vi "FPGA1483V1_0.vi"() -> ()   [LabVIEW 2013]
doc: "This is the FPGA VI for the 10-Tap 8-Bit Camera with DRAM example. This example demonstrates how to acquire images from a 10-tap, 8-bit, extended configuration, Camera Link camera and transfer the images to the host. This example supports area scan and line scan cameras for both continuous and finite acquisitions.\n\nThis example also demonstrates the use of DRAM as a frame buffer for very high speed acquisitions. Data packing and flow-control are also employed to maximize use of the available DRAM and FIFOs in terms of both memory space and performance.\n\nAdditionally, the example demonstrates the serial server, which allows third-party camera configuration utilities to communicate with the camera using the Camera Link serial interface while this VI is running."
uses:
  <vilib>/Platform/TimedLoop/XDataNode/timing_clust.ctl
  <vilib>/Platform/TimedLoop/XDataNode/nitl_modes.ctl
  <vilib>/Platform/TimedLoop/XDataNode/wakeup.ctl
  <vilib>/rvi/eio/common/nirviEmuTemplateMethod_errors.vi
  <vilib>/rvi/Emulation/niFpgaSctlEmulationGetInTimedLoop.vi
  <vilib>/rvi/Emulation/niFpgaEmulationReportErrorSimple.vi
  <vilib>/rvi/Emulation/niFpgaGetClockAttributes.vi
  <vilib>/rvi/Emulation/niFpgaCriticalErrorInLSC.vi
  Common/CL Data to Pixels/10 Tap 8-Bit.vi
  <vilib>/rvi/interface/RandomDataEmulation/nirviRandomDataFPGAFIFO.vi
  <vilib>/rvi/interface/RandomDataEmulation/niFpgaRandomDataHandleErrors.vi
  <vilib>/rvi/FIFO/Fifo_Resource/nirvififoEmulationWriteFpgaImpl.vi
  <vilib>/rvi/DataTransferAndStorage/Container/Common/niFpgaContainerGetUniqueNameForEmu.vi
  <vilib>/rvi/FIFO/Fifo_Resource/nirvififoEmulationGetNumberOfElementsToReadFpgaImpl.vi
  <vilib>/rvi/FIFO/Fifo_Resource/nirvififoEmulationReadFpgaImpl.vi
  <vilib>/rvi/Emulation/niFpgaProcessEmulError.vi
  <vilib>/Platform/TimedLoop/XDataNode/XDataNode.xnode
  <vilib>/eio/EIONode/EIONode.xnode
  <vilib>/rvi/DataTransferAndStorage/Container/XNode/niFpgaContainer.xnode
  <vilib>/rvi/interface/RandomDataEmulation/nirviRandomDataFpgaReadWriteTemplate.vi
  <vilib>/rvi/FIFO/Fifo_Resource/nirvififoEmulationWrite.vi
  <vilib>/rvi/FIFO/Fifo_Resource/nirvififoEmulationGetNumberOfElementsToRead.vi
  <vilib>/rvi/FIFO/Fifo_Resource/nirvififoEmulationRead.vi
  <vilib>/Platform/TimedLoop/XDataNode/XDNodeRunTimeDep.lvlib
panel:
  in  "DigitalEnable":bool=TRUE
  out "auxAI1":i16
  in  "auxAO0":i16
  out "auxAI0":i16
  out "DI1":bool
  out "DI0":bool
  in  "DO1":bool
  in  "DO0":bool
  out "DevQualityStatus":u8
  out "DMAsOverflow":u16
  out "BytesperSampleChannelDMATtoHOST":u8[](array[numeric])=[12]
  out "FrameTypeDMATtoHOST":u8[](array[numeric])=[12]
  out "Platform":enum8{"FlexRIO", "cRIO", "RSeries"}(ring)
  in  "GroupEnable0":bool
  out "DMAsOverflowB":bool
  out "DevProfile":u8=1
  out "RIOAdapterCorrect":bool
  out "InsertedIOModule ID":u32=278099145
  out "ExpectedIOModule ID":u32=278099145
  in  "DebugMode":bool
  in  "SamplingRate0":u16
  out "DeviceTemp":i16=147
  in  "DataBytetoTx":i32=1 format="%x"
  in  "DAQStartStop":bool
  out "NCHperDMATtoHOST":u8[](array[numeric])=[1]
  out "FPGAVIversion":u8[](array[numeric])=[1, 1]
  out "NoOfWFGen":u8
  out "Fref":u32=100000000
  in  "ControlEnable":bool=TRUE caption="IO Module\\CL Control Enable"
  in  "Configuration":u8=2 caption="CL Config.Configuration"
  in  "SignalMapping":u8 caption="CL Config.Signal Mapping"
  in  "LineScan":bool caption="CL Config.Line Scan"
  in  "DVALHigh":bool=TRUE caption="CL Config.DVAL Active High"
  in  "LVALHigh":bool=TRUE caption="CL Config.LVAL Active High"
  in  "FVALHigh":bool=TRUE caption="CL Config.FVAL Active High"
  in  "SpareHigh":bool=TRUE caption="CL Config.Spare Active High"
  in  "Acq Control.Line Scan Height":u32
  in  "Acq Control.Frames To Acq":u32
  in  "StartDAQ":bool
  in  "StopDAQ":bool
  in  "Acq Control.Ignore DVAL":bool
  out "Acq Status.Acq In Progress":bool
  out "Acq Status.Clocks Per Line":u32
  out "Acq Status.Frames Acq'd":u32
  out "Acq Status.Lines Per Frame":u32
  out "auxDO11":bool caption="Acq Status.DMA Write Timeout"
  out "InitDone":bool
  in  "uartBaudRate":i32=1 caption="UART.Baud Rate"
  in  "uartTransmit":bool caption="UART.Transmit"
  in  "uartSetBaudRate":bool caption="UART.Set Baud Rate"
  in  "uartByteMode":bool=TRUE caption="UART.Byte Mode"
  out "uartRxReady":bool caption="auxDI1"
  out "uartBreakIndicator":bool caption="UART.Break Indicator"
  out "uartFramingError":bool caption="UART.Framing Error"
  out "uartOverrunError":bool caption="UART.Overrun Error"
  out "uartTxReady":bool caption="UART.Tx Ready"
  out "uartRxData":i32 caption="UART.Rx Data" format="%02x"
  in  "uartReceive":bool caption="UART.Receive"
  # "This terminal has not sense in this solution"
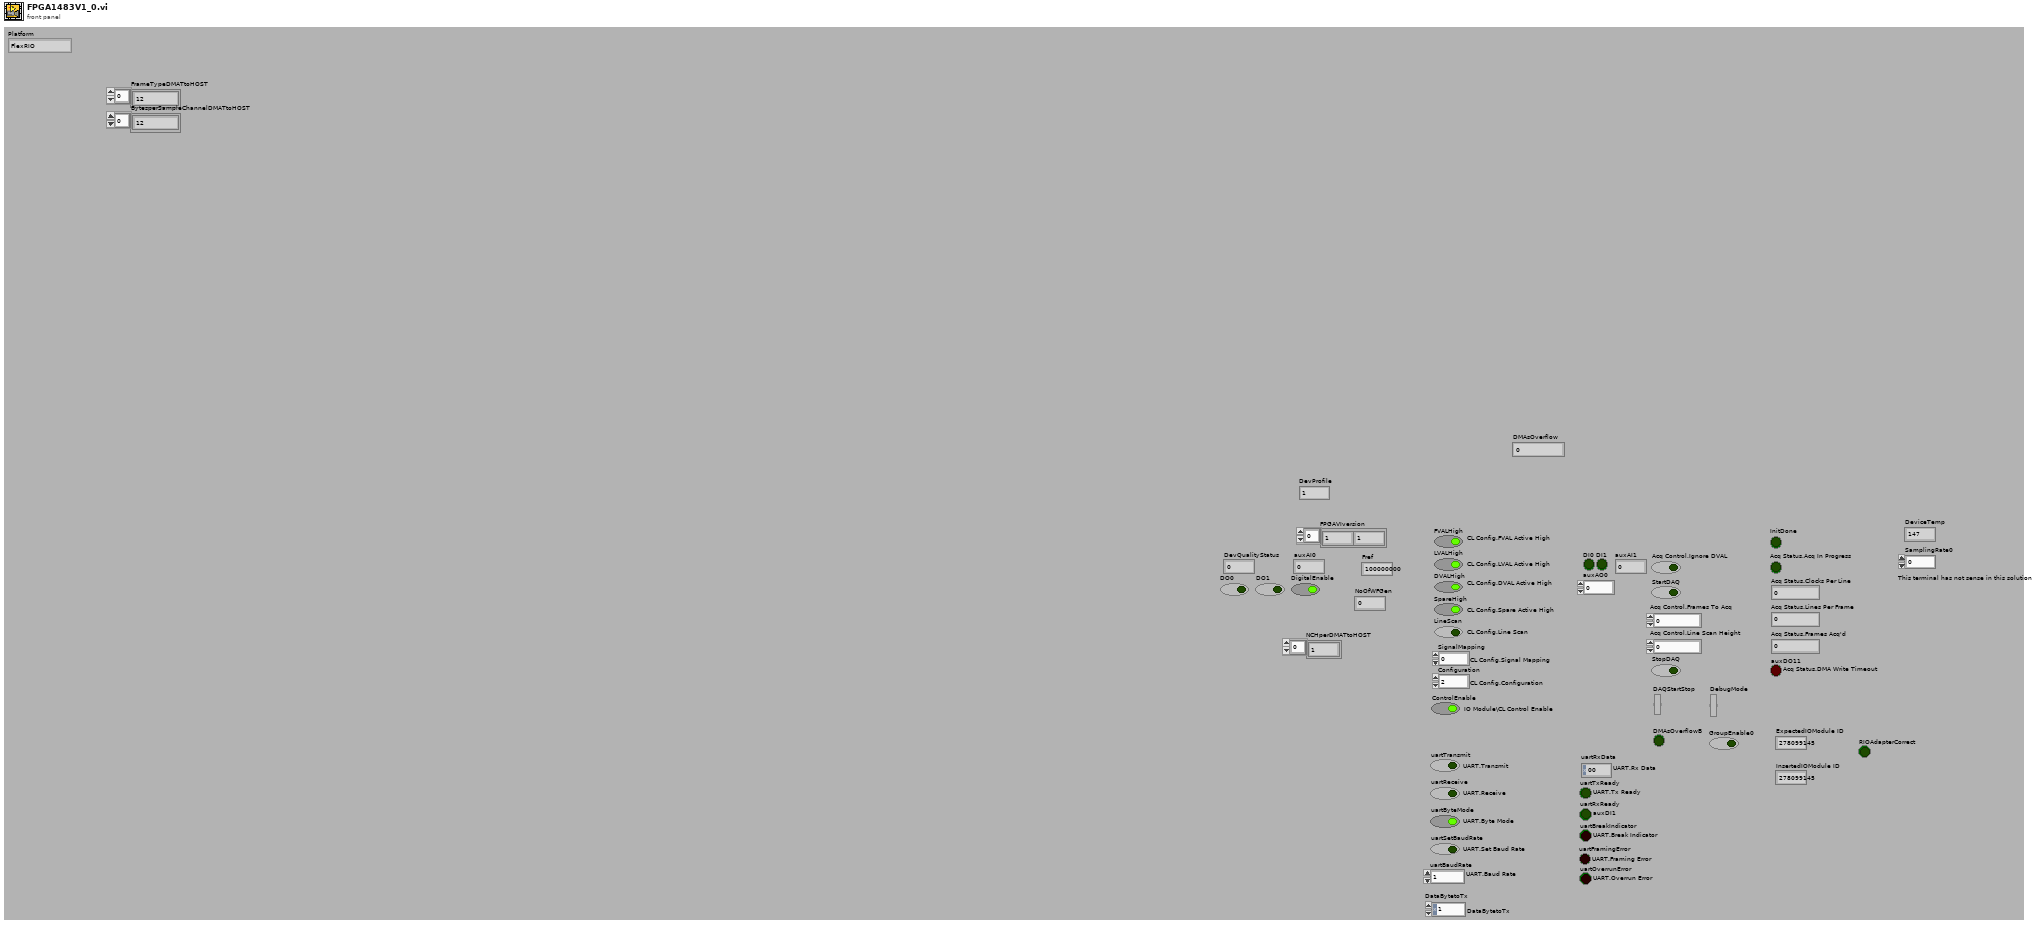
[diagram p1: front panel]
types:
  T1 = typedef "XDNodeRunTimeDep.lvlib/timing_clust.ctl" = cluster{"Expected End [f-1]":u64, "Actual End [f-1]":u64, "Finished Late? [f-1]":bool, "Expected End [i-1]":u64, "Actual End [i-1]":u64, "Finished Late? [i-1]":bool, "Expected Start [i]":u64, "Actual Start [i]":u64, "Expected Start [f]":u64, "Actual Start [f]":u64, "Source Name":string, "Structure Name":string, "Period":i64, "Deadline":i64, "Offset":i64, "Start":i64, "Priority":i32, "Timeout":i32, "Mode":T2, "Wakeup Reason":T3, "Error":errorcluster, "Source Type":string, "Secondary Source Type":string, "Global End Time":u64, "Global Start Time":u64, "Frame Duration":u64, "Iteration Duration":u64, "Assigned CPU":i32, "I/O Scan Engine Mode":u32}
  T2 = typedef "XDNodeRunTimeDep.lvlib/nitl_modes.ctl" = enum32{"No Change", "Process missed periods, maintain original phase", "Discard missed periods, maintain original phase", "Process missed periods, ignore original phase", "Discard missed periods, ignore original phase"}
  T3 = typedef "XDNodeRunTimeDep.lvlib/wakeup.ctl" = enum32{"Normal", "Aborted", "Asynchronous wakeup", "Timing source error", "Timed loop error", "Timeout"}
  T4 = cluster{"Enables Valid":bool, "Frame Valid":bool, "Line Valid":bool, "Data Valid":bool}
  T5 = enum8{"Standard", "Basler 10-tap", "Vosskühler 10-tap"}
  T6 = cluster{"Pixel 0":u8, "Pixel 1":u8, "Pixel 2":u8, "Pixel 3":u8, "Pixel 4":u8, "Pixel 5":u8, "Pixel 6":u8, "Pixel 7":u8, "Pixel 8":u8, "Pixel 9":u8}
  T7 = cluster{"Tx Data":u8[], "Transmit":bool, "Receive":bool, "Byte Mode":bool, "Set Baud Rate":bool, "Baud Rate":u8}
  T8 = cluster{"Rx Data":u8, "Turn Off Transmit":bool, "Turn Off Receive":bool, "Turn Off Set Baud Rate":bool, "Tx Ready":bool, "Rx Ready":bool, "Break Indicator":bool, "Framing Error":bool, "Overrun Error":bool}
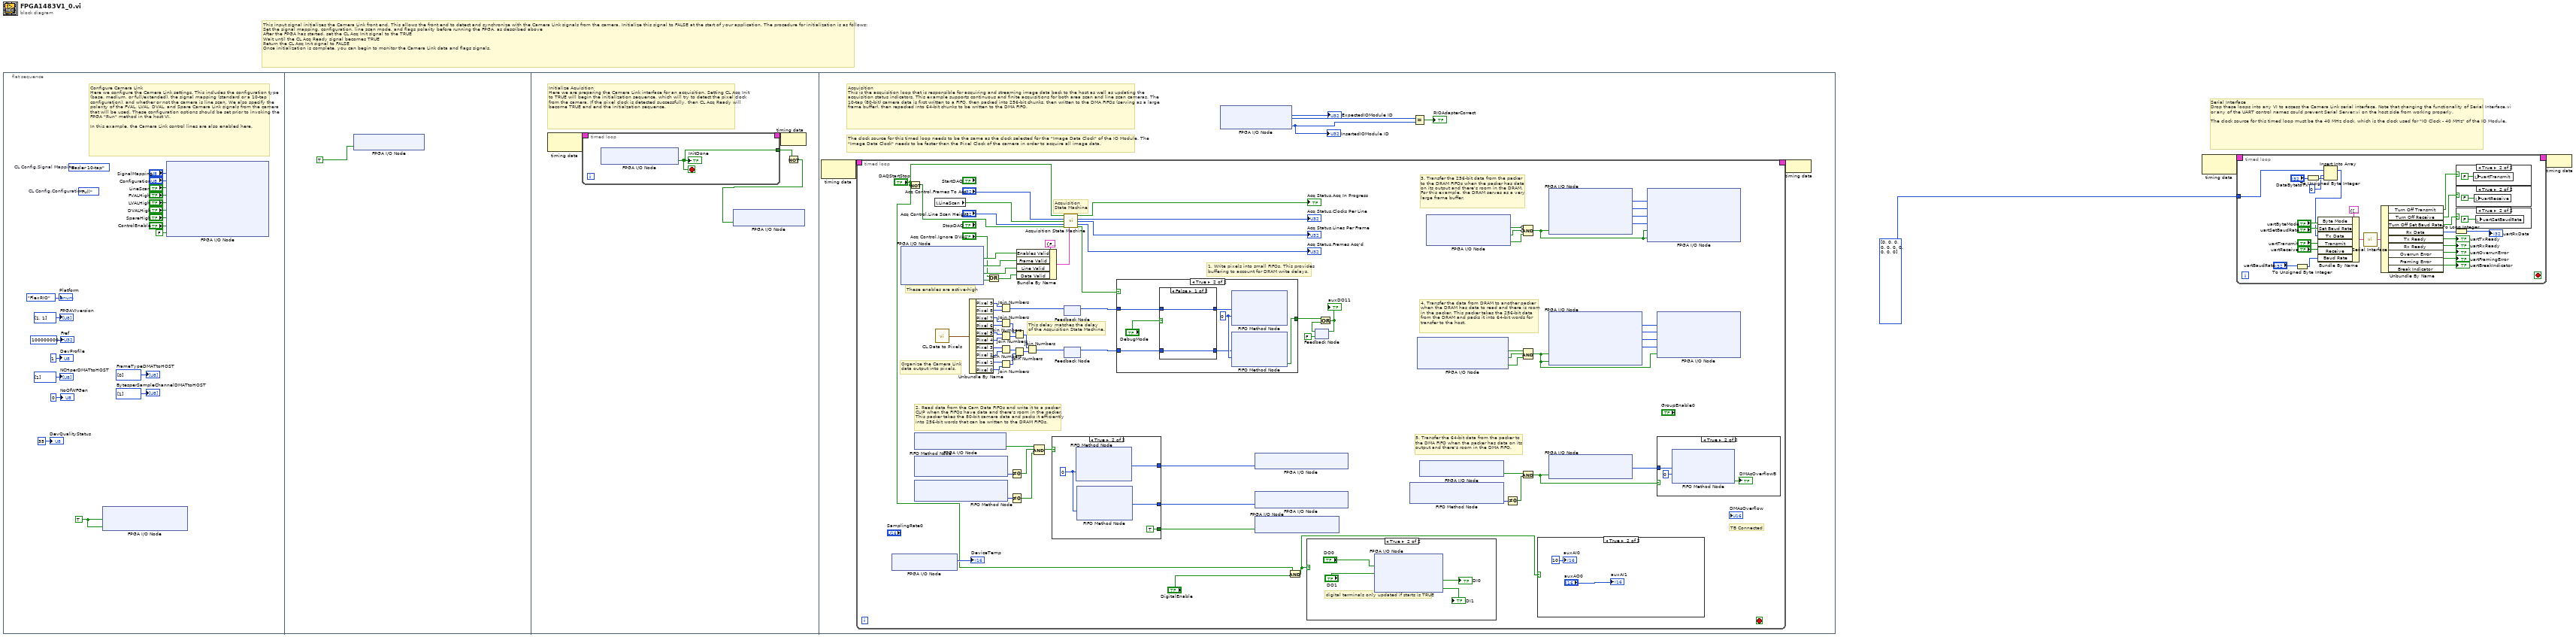
[diagram p0: block diagram]
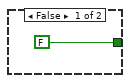
[diagram p9: hidden frame]
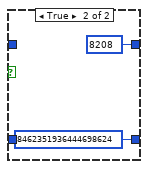
[diagram p10: hidden frame]
diagram:
  # "This input signal initializes the Camera Link front end. This allows the front end to detect and synchronize with the Camera Link signals from the camera. Initialize this signal to FALSE at the start of your application. The procedure for initialization is as follows: \nSet the signal mapping, configuration, line scan mode, and flags polarity before running the FPGA, as described above \nAfter the FPGA has started, set the CL Acq Init signal to the TRUE \nWait until the CL Acq Ready signal becomes TRUE \nReturn the CL Acq Init signal to FALSE \nOnce initialization is complete, you can begin to monitor the Camera Link data and flags signals."
  # "Serial Interface\nDrop these loops into any VI to access the Camera Link serial interface. Note that changing the functionality of Serial Interface.vi or any of the UART control names could prevent Serial Server.vi on the host side from working properly.\n\nThe clock source for this timed loop must be the 40 MHz clock, which is the clock used for \"IO Clock - 40 MHz\" of the IO Module."
  n1 = flat-sequence {
    frame #0 {
      w4 = TRUE ("IO Module\\TTL Out Enable 0")
      (unwired) T5."Basler 10-tap"  # CL Config.Signal Mapping
      (unwired) enum8{"Base", "Medium", "Full"}."Full"  # CL Config.Configuration
      # "Configure Camera Link\nHere we configure the Camera Link settings. This includes the configuration type (base, medium, or full/extended), the signal mapping (standard or a 10-tap configuration), and whether or not the camera is line scan. We also specify the polarity of the FVAL, LVAL, DVAL, and Spare Camera Link signals from the camera that will be used. These configuration options should be set prior to invoking the FPGA \"Run\" method in the host VI.\n\nIn this example, the Camera Link control lines are also enabled here."
      n2 = xnode "FPGA I/O Node"("IO Module\\TTL Out Enable 0"=w4, "IO Module\\TTL Out Enable 1"=w4) -> ()  [unwired: 2 in, 2 out]
      n3 = xnode "FPGA I/O Node"("IO Module\\CL Set Signal Mapping"="SignalMapping", "IO Module\\CL Set Configuration"="Configuration", "IO Module\\CL Set Line Scan"="LineScan", "IO Module\\CL Set FVAL Active High"="FVALHigh", "IO Module\\CL Set LVAL Active High"="LVALHigh", "IO Module\\CL Set DVAL Active High"="DVALHigh", "IO Module\\CL Set Spare Active High"="SpareHigh", "IO Module\\CL Control Enable"="ControlEnable", "IO Module\\CL Acq Init"=FALSE ("IO Module\\CL Acq Init")) -> ()  [unwired: 9 in, 9 out]
      "Fref" <- u32 100000000 ("Fref")
      "NoOfWFGen" <- u8 0 ("NoOfWFGen")
      "FPGAVIversion" <- u8[] [1, 1] ("FPGAVIversion")
      "NCHperDMATtoHOST" <- u8[] [1] ("NCHperDMATtoHOST")
      "DevProfile" <- u8 1 ("DevProfile")
      "Platform" <- enum8{"FlexRIO", "cRIO", "RSeries"}."FlexRIO" ("Platform")
      "FrameTypeDMATtoHOST" <- u8[] [0]
      "BytesperSampleChannelDMATtoHOST" <- u8[] [1]
      "DevQualityStatus" <- u8 35 ("DevQualityStatus")
    }
    frame #1 {
      n4 = xnode "FPGA I/O Node"("IO Module\\CL Acq Init"=TRUE) -> ()  [unwired: 1 in, 1 out]
    }
    frame #2 {
      # "Initialize Aquisition\nHere we are preparing the Camera Link interface for an acquisition. Setting CL Acq Init to TRUE will begin the initialization sequence, which will try to detect the pixel clock from the camera. If the pixel clock is detected successfully, then CL Acq Ready will become TRUE and end the initialzation sequence."
      n5 = node-c288() -> (w27:T1)  [unwired: 1 out]
      n6 = timed-loop {
        timing: w27 -> [_]
        timing-out: [_] -> w26
        tunnel: [w28] -> w25
        stop <- w28 stop-if-true
        n7 = xnode "FPGA I/O Node"() -> ("IO Module\\CL Acq Ready"=w28:bool)  [unwired: 1 in, 1 out]
        "InitDone" <- w28
      }
      n8 = node-c288(w26) -> ()
      n9 = Not(x=w25) -> (.not. x?=w24:bool)
      n10 = xnode "FPGA I/O Node"("IO Module\\CL Acq Init"=w24) -> ()  [unwired: 1 in, 1 out]
    }
    frame #3 {
      # "The clock source for this timed loop needs to be the same as the clock selected for the \"Image Data Clock\" of the IO Module. The \"Image Data Clock\" needs to be faster than the Pixel Clock of the camera in order to acquire all image data."
      # "Acquisition\nThis is the acquisition loop that is responsible for acquiring and streaming image data back to the host as well as updating the acquisition status indicators. This example supports continuous and finite acquisitions for both area scan and line scan cameras. The 10-tap (80-bit) camera data is first written to a FIFO, then packed into 256-bit chunks, then written to the DMA FIFOs (serving as a large frame buffer), then repacked into 64-bit chunks to be written to the DMA FIFO."
      n11 = node-c288() -> (w37:T1)  [unwired: 1 in]
      n12 = timed-loop {
        timing: w37 -> [_]
        timing-out: [_] -> w36
        stop <- _ stop-if-true
        # "TB Connected"
        # "3. Transfer the 256-bit data from the packer\nto the DRAM FIFOs when the packer has data\non its output and there's room in the DRAM.\nFor this example, the DRAM serves as a very\nlarge frame buffer."
        # "5. Transfer the 64-bit data from the packer to\nthe DMA FIFO when the packer has data on its\noutput and there's room in the DMA FIFO."
        # "4. Transfer the data from DRAM to another packer\nwhen the DRAM has data to read and there is room\nin the packer. This packer takes the 256-bit data\nfrom the DRAM and packs it into 64-bit words for\ntransfer to the host."
        # "2. Read data from the Cam Data FIFOs and write it to a packer\nCLIP when the FIFOs have data and there's room in the packer.\nThis packer takes the 80-bit camera data and packs it efficiently\ninto 256-bit words that can be written to the DRAM FIFOs."
        # "1. Write pixels into small FIFOs. This provides\nbuffering to account for DRAM write delays."
        # "Organize the Camera Link\ndata output into pixels."
        # "These enables are active-high"
        # "This delay matches the delay\nof the Acquisition State Machine."
        # "Acquisition\nState Machine"
        n13 = xnode "FPGA I/O Node"() -> ("Device Temperature"=→"DeviceTemp":i16)  [unwired: 1 in, 1 out]
        n14 = xnode "FPGA I/O Node"() -> ("IO Module\\CL Output Valid"=w101:bool, "IO Module\\CL Frame Valid"=w100:bool, "IO Module\\CL Line Valid"=w99:bool, "IO Module\\CL Data Valid"=w96:bool)  [unwired: 4 in, 4 out]
        n15 = Not(x="DAQStartStop") -> (.not. x?=w42:bool)
        n16 = xnode "FPGA I/O Node"() -> ("Pack 80 To 256\\Ready For Write"=w67:bool)  [unwired: 1 in, 1 out]
        n17 = xnode ("FIFO Method Node")() -> ("Number of Elements to Read"=w71:u32)  [unwired: 1 in, 1 out]
        n18 = xnode ("FIFO Method Node")() -> ("Number of Elements to Read"=w70:u32)  [unwired: 1 in, 1 out]
        n19 = local read "LineScan"() -> (w93:bool)
        n20 = call-poly "CL Data to Pixels.vi"() -> ("Pixels"=w113:T6)  [unwired: 1 in]
        n21 = Unbundle By Name(w113) -> ("Pixel 9"=w91:u8, "Pixel 8"=w90:u8, "Pixel 7"=w89:u8, "Pixel 6"=w88:u8, "Pixel 5"=w87:u8, "Pixel 4"=w86:u8, "Pixel 3"=w85:u8, "Pixel 2"=w84:u8, "Pixel 1"=w83:u8, "Pixel 0"=w82:u8)
        n22 = Or(x="Acq Control.Ignore DVAL", y=w96) -> (x .or. y?=w95:bool)
        n23 = Join Numbers(hi=w91, lo=w90) -> ((hi.lo)=w77:u16)
        n24 = Join Numbers(hi=w89, lo=w88) -> ((hi.lo)=w80:u16)
        n25 = Join Numbers(hi=w87, lo=w86) -> ((hi.lo)=w79:u16)
        n26 = Join Numbers(hi=w85, lo=w84) -> ((hi.lo)=w78:u16)
        n27 = Join Numbers(hi=w83, lo=w82) -> ((hi.lo)=w81:u16)
        n28 = Not Equal To 0?(x=w71) -> (x != 0?=w65:bool)
        n29 = Not Equal To 0?(x=w70) -> (x != 0?=w64:bool)
        n30 = Join Numbers(hi=w80, lo=w79) -> ((hi.lo)=w76:u32)
        n31 = Join Numbers(hi=w78, lo=w81) -> ((hi.lo)=w75:u32)
        n32 = Bundle By Name(cluster=T4 {"Enables Valid"=FALSE, "Frame Valid"=FALSE, "Line Valid"=FALSE, "Data Valid"=FALSE} ("Enables"), "Enables Valid"=w101, "Frame Valid"=w100, "Line Valid"=w99, "Data Valid"=w95) -> (w98:T4)
        n33 = Join Numbers(hi=w76, lo=w75) -> ((hi.lo)=w74:u64)
        n34 = Compound Arithmetic op=AND(w67, w65, w64) -> (w66:bool)
        n35 = case shown="True" w66 {
          tunnel: [_ w126] -> w72
          tunnel: [_ w125] -> w68
          tunnel: [_ TRUE] -> w69
          frame False {
          }
          frame True {
            w124 = 0 ("Timeout")
            n36 = xnode ("FIFO Method Node")("Timeout"=w124) -> ("Element"=w126:u16)  [unwired: 1 in, 2 out]
            n37 = xnode ("FIFO Method Node")("Timeout"=w124) -> ("Element"=w125:u64)  [unwired: 1 in, 2 out]
          }
        }
        n38 = call "Acquisition State Machine.vi"("Acquire"="DAQStartStop", "Frames to Acquire"="Acq Control.Frames To Acq", "Line Scan"=w93, "Line Scan Height"="Acq Control.Line Scan Height", "Cancel Acq"=w42, "Enables"=w98) -> ("Acq In Progress"=→"Acq Status.Acq In Progress":bool, "Num Clocks Per Line"=→"Acq Status.Clocks Per Line":u32, "Num Lines Per Frame"=→"Acq Status.Lines Per Frame":u32, "Num Frames Acq'd"=→"Acq Status.Frames Acq'd":u32, "Capture Cycle"=w111:bool)  [unwired: 4 in, 1 out]
        n39 = feedback #1() -> (w73:u16)  [unwired: 1 in]
        n40 = feedback-in #1(w77) -> ()
        n41 = feedback-in #2(w74) -> ()
        n42 = feedback #2() -> (w112:u64)  [unwired: 1 in]
        n43 = case shown="True" w111 {
          tunnel: [FALSE ("Timed Out?") w134] -> w109
          tunnel: w112 -> [_ w129]
          tunnel: w73 -> [_ w131]
          frame False {
          }
          frame True {
            w133 = 0 ("Timeout")
            n44 = case shown="False" "DebugMode" {
              tunnel: w131 -> [w136 _]
              tunnel: [w136 u16 8208] -> w130
              tunnel: w129 -> [w135 _]
              tunnel: [w135 u64 8462351936444698624] -> w128
              frame False {
              }
              frame True {
              }
            }
            n45 = xnode ("FIFO Method Node")("Element"=w130, "Timeout"=w133) -> ()  [unwired: 1 in, 2 out]
            n46 = xnode ("FIFO Method Node")("Element"=w128, "Timeout"=w133) -> ("Timed Out?"=w134:bool)  [unwired: 1 in, 1 out]
          }
        }
        n47 = xnode "FPGA I/O Node"("Pack 80 To 256\\Data In Upper 16"=w72) -> ()  [unwired: 1 in, 1 out]
        n48 = xnode "FPGA I/O Node"("Pack 80 To 256\\Data In Lower 64"=w68) -> ()  [unwired: 1 in, 1 out]
        n49 = xnode "FPGA I/O Node"("Pack 80 To 256\\Write Enable"=w69) -> ()  [unwired: 1 in, 1 out]
        n50 = And(x="DAQStartStop", y="DigitalEnable") -> (x .and. y?=w38:bool)
        n51 = case shown="True" w38 {
          frame False {
          }
          frame True {
            # "digital terminals only updated if starts is TRUE"
            n52 = xnode "FPGA I/O Node"("IO Module\\TTL Out 0"="DO0", "IO Module\\TTL Out 1"="DO1") -> ("IO Module\\TTL In 2"=→"DI0":bool, "IO Module\\TTL In 3"=→"DI1":bool)  [unwired: 4 in, 4 out]
          }
        }
        n53 = feedback #3(FALSE) -> (w108:bool)
        n54 = Or(x=w109, y=w108) -> (x .or. y?=w107:bool)
        "auxDO11" <- w107
        n55 = feedback-in #3(w107) -> ()
        n56 = xnode ("FIFO Method Node")() -> ("Number of Elements to Write"=w53:u32)  [unwired: 1 in, 1 out]
        n57 = xnode "FPGA I/O Node"() -> ("DRAM Bank 1\\Data_Available"=w63:bool, "DRAM Bank 0\\Data_Available"=w61:bool, "Pack 256 To 64\\Ready for Write"=w62:bool)  [unwired: 3 in, 3 out]
        n58 = xnode "FPGA I/O Node"() -> ("Pack 256 To 64\\Output Valid"=w55:bool)  [unwired: 1 in, 1 out]
        n59 = xnode "FPGA I/O Node"() -> ("DRAM Bank 1\\Full"=w47:bool, "DRAM Bank 0\\Full"=w48:bool, "Pack 80 To 256\\Output Valid"=w44:bool)  [unwired: 3 in, 3 out]
        n60 = Not Equal To 0?(x=w53) -> (x != 0?=w54:bool)
        n61 = And(x=w55, y=w54) -> (x .and. y?=w43:bool)
        n62 = Compound Arithmetic op=AND(invert w47, invert w48, w44) -> (w46:bool)
        n63 = Compound Arithmetic op=AND(w63, w61, w62) -> (w45:bool)
        n64 = case shown="True" w38 {
          frame False {
          }
          frame True {
            "auxAI0" <- i16 10 ("auxAI0")
            "auxAI1" <- "auxAO0"
          }
        }
        n65 = xnode "FPGA I/O Node"("Pack 80 To 256\\Read Enable"=w46) -> ("Pack 80 To 256\\Data Out 3"=w49:u64, "Pack 80 To 256\\Data Out 2"=w50:u64, "Pack 80 To 256\\Data Out 1"=w52:u64, "Pack 80 To 256\\Data Out 0"=w51:u64)  [unwired: 5 in, 5 out]
        n66 = xnode "FPGA I/O Node"("DRAM Bank 1\\Read"=w45, "DRAM Bank 0\\Read"=w45) -> ("DRAM Bank 1\\Read_Data_Upper"=w59:u64, "DRAM Bank 1\\Read_Data_Lower"=w58:u64, "DRAM Bank 0\\Read_Data_Upper"=w57:u64, "DRAM Bank 0\\Read_Data_Lower"=w56:u64)  [unwired: 6 in, 6 out]
        n67 = xnode "FPGA I/O Node"("Pack 256 To 64\\Read Enable"=w43) -> ("Pack 256 To 64\\Data Out 64"=w60:u64)  [unwired: 2 in, 2 out]
        n68 = xnode "FPGA I/O Node"("DRAM Bank 1\\Write_Data_Upper"=w49, "DRAM Bank 1\\Write_Data_Lower"=w50, "DRAM Bank 0\\Write_Data_Upper"=w52, "DRAM Bank 0\\Write_Data_Lower"=w51, "DRAM Bank 1\\Write"=w46, "DRAM Bank 0\\Write"=w46) -> ()  [unwired: 6 in, 6 out]
        n69 = xnode "FPGA I/O Node"("Pack 256 To 64\\Data In 3"=w59, "Pack 256 To 64\\Data In 2"=w58, "Pack 256 To 64\\Data In 1"=w57, "Pack 256 To 64\\Data In 0"=w56, "Pack 256 To 64\\Write Enable"=w45) -> ()  [unwired: 5 in, 5 out]
        n70 = case shown="True" w43 {
          tunnel: w60 -> [_ w122]
          frame False {
          }
          frame True {
            n71 = xnode ("FIFO Method Node")("Element"=w122, "Timeout"=0) -> ("Timed Out?"=→"DMAsOverflowB":bool)  [unwired: 1 in, 1 out]
          }
        }
      }
      n72 = xnode "FPGA I/O Node"() -> ("Expected IO Module ID"=w35:u32, "Inserted IO Module ID"=w34:u32)  [unwired: 2 in, 2 out]
      "ExpectedIOModule ID" <- w35
      "InsertedIOModule ID" <- w34
      n73 = Equal?(x=w35, y=w34) -> (x = y?=→"RIOAdapterCorrect":bool)
      n74 = node-c288(w36) -> ()
    }
  }
  n75 = node-c288() -> (w3:T1)  [unwired: 1 out]
  n76 = timed-loop {
    timing: w3 -> [_]
    timing-out: [_] -> w2
    tunnel: u8[] [0, 0, 0, 0, 0, 0, 0, 0, 0, 0] -> [w148]
    stop <- _ stop-if-true
    n77 = To Unsigned Byte Integer(number="uartBaudRate") -> (unsigned 8bit integer=w145:u8)
    n78 = To Unsigned Byte Integer(number="DataBytetoTx") -> (unsigned 8bit integer=w151:u8)
    n79 = Insert Into Array(array=w148, index=0, new element=w151) -> (w147:u8[])
    n80 = Bundle By Name(cluster=T7 {"Tx Data"=[0, 0, 0, 0, 0, 0, 0, 0, 0, 0], "Transmit"=FALSE, "Receive"=FALSE, "Byte Mode"=TRUE, "Set Baud Rate"=FALSE, "Baud Rate"=0} ("UART Inputs"), "Byte Mode"="uartByteMode", "Set Baud Rate"="uartSetBaudRate", "Tx Data"=w147, "Transmit"="uartTransmit", "Receive"="uartReceive", "Baud Rate"=w145) -> (w152:T7)
    n81 = call "Serial Interface.vi"("UART Inputs"=w152) -> ("UART Outputs"=w162:T8)
    n82 = Unbundle By Name(w162) -> ("Turn Off Transmit"=w155:bool, "Turn Off Receive"=w156:bool, "Turn Off Set Baud Rate"=w154:bool, "Rx Data"=w143:u8, "Tx Ready"=→"uartTxReady":bool, "Rx Ready"=→"uartRxReady":bool, "Overrun Error"=→"uartOverrunError":bool, "Framing Error"=→"uartFramingError":bool, "Break Indicator"=→"uartBreakIndicator":bool)
    n83 = To Long Integer(number=w143) -> (32bit integer=→"uartRxData":i32)
    n84 = case shown="True" w155 {
      frame False {
      }
      frame True {
        n85 = local write "uartTransmit"(FALSE ("UART.Transmit")) -> ()
      }
    }
    n86 = case shown="True" w156 {
      frame False {
      }
      frame True {
        n87 = local write "uartReceive"(FALSE ("UART.Receive")) -> ()
      }
    }
    n88 = case shown="True" w154 {
      frame False {
      }
      frame True {
        n89 = local write "uartSetBaudRate"(FALSE ("UART.Receive")) -> ()
      }
    }
  }
  n90 = node-c288(w2) -> ()
